vi "E15_State_Mach_Coins.vi"() -> ()   [LabVIEW 2020]
panel:
  out "Dinero Depositado":string
  out "Despachar":bool
  in  "10 cents":bool
  in  "5 cents":bool
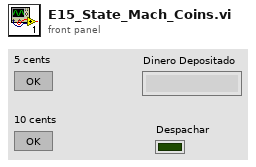
[diagram p1: front panel]
types:
  T1 = enum16{"Inicio", "5 Cents", "10 Cents", "Despacho"}
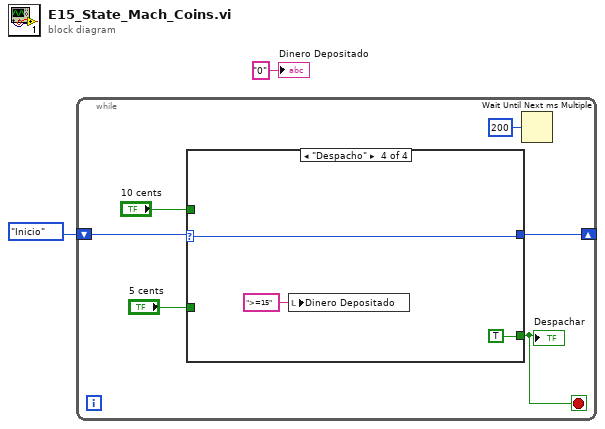
[diagram p0: block diagram]
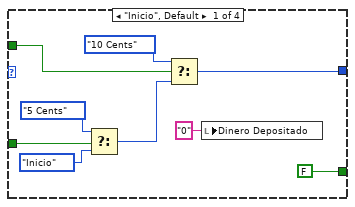
[diagram p2: hidden frame]
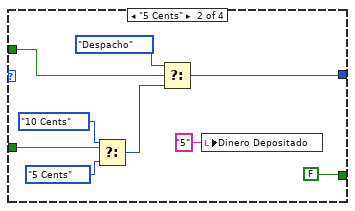
[diagram p3: hidden frame]
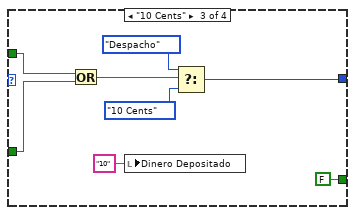
[diagram p4: hidden frame]
diagram:
  n1 = while {
    shift-right: [w5] -> _
    shift-left: T1."Inicio" -> [w8]
    stop <- w3 stop-if-true
    n2 = case shown="\"Despacho\"" w8 {
      selector: w8 -> [_ _ _ w35]
      tunnel: "5 cents" -> [w17 w25 w33 _]
      tunnel: "10 cents" -> [w11 w26 w34 _]
      tunnel: [w12 w20 w29 w35] -> w5
      tunnel: [FALSE FALSE FALSE TRUE] -> w3
      frame "Inicio", Default {
        n3 = Select(t=T1."5 Cents", s=w17, f=T1."Inicio") -> (s? t:f=w13:T1)
        n4 = Select(t=T1."10 Cents", s=w11, f=w13) -> (s? t:f=w12:T1)
        n5 = local write "Dinero Depositado"("0" ("Dinero Depositado")) -> ()
      }
      frame "5 Cents" {
        n6 = Select(t=T1."10 Cents", s=w25, f=T1."5 Cents") -> (s? t:f=w22:T1)
        n7 = Select(t=T1."Despacho", s=w26, f=w22) -> (s? t:f=w20:T1)
        n8 = local write "Dinero Depositado"("5" ("Dinero Depositado")) -> ()
      }
      frame "10 Cents" {
        n9 = Or(x=w34, y=w33) -> (x .or. y?=w32:bool)
        n10 = local write "Dinero Depositado"("10" ("Dinero Depositado")) -> ()
        n11 = Select(t=T1."Despacho", s=w32, f=T1."10 Cents") -> (s? t:f=w29:T1)
      }
      frame "Despacho" {
        n12 = local write "Dinero Depositado"(">=15" ("Dinero Depositado")) -> ()
      }
    }
    "Despachar" <- w3
    n13 = Wait Until Next ms Multiple(millisecond multiple=u32 200) -> ()  [unwired: 1 out]
  }
  "Dinero Depositado" <- "0" ("Dinero Depositado")
